vi "插入数据.vi"(8 "error in (no error)":errorcluster, 9 "SQL query":string, 11 "sqlerver in":refnum<class "sqlerver.lvclass">) -> (0 "error out":errorcluster, 3 "sqlerver out":refnum<class "sqlerver.lvclass">)   [LabVIEW 2016, in "sqlerver.lvclass"]
uses:
  sqlerver.lvclass
  sqlerver.lvclass/sqlerver.ctl
  <vilib>/addons/database/Connection.llb/Conn Execute.vi
  <vilib>/addons/database/Recordset.llb/Rec Destroy - Connection.vi
  <vilib>/addons/database/NI_Database_API.lvlib
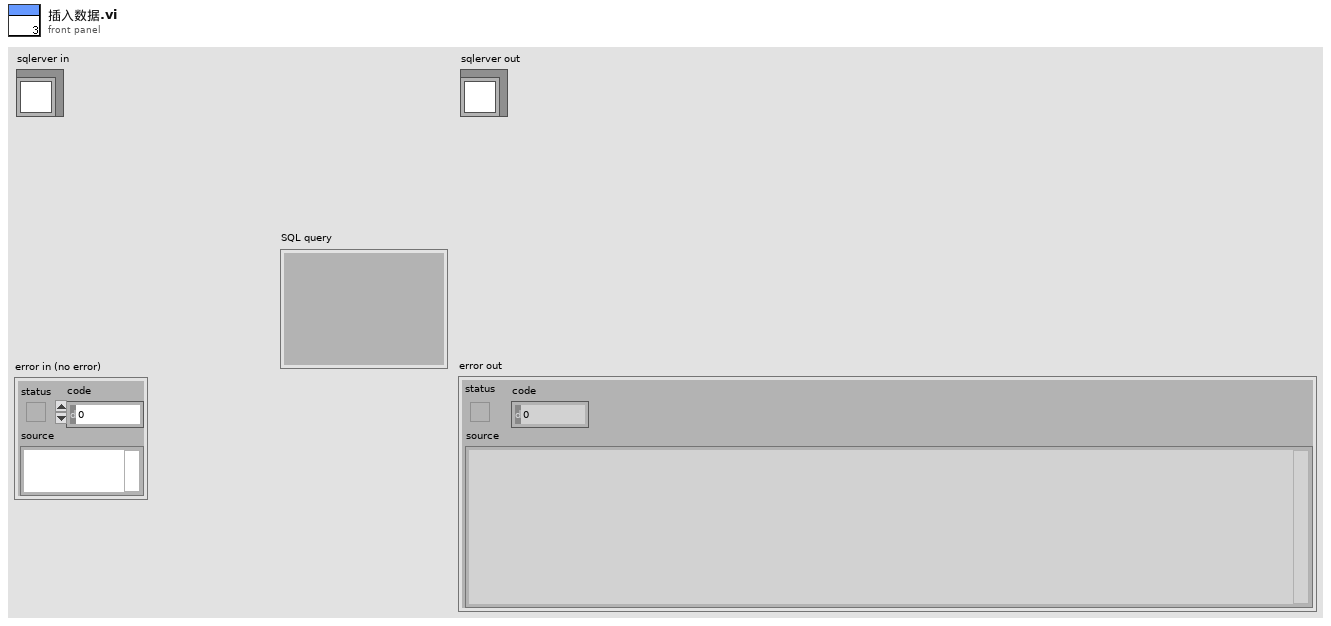
[diagram p1: front panel]
types:
  T1 = typedef "NI_Database_API.lvlib/Conn ObjectReference.ctl" = refnum<k1>
  T2 = typedef "NI_Database_API.lvlib/Rec ObjectReference.ctl" = refnum<k1>
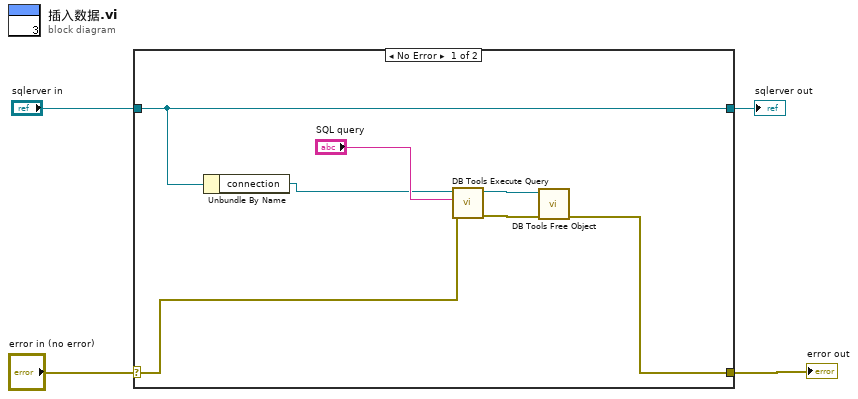
[diagram p0: block diagram]
diagram:
  n1 = case shown="No Error" "error in (no error)" {
    selector: "error in (no error)" -> [w8 w13]
    tunnel: [w7 w13] -> w3
    tunnel: [w6 w12] -> w1
    tunnel: "sqlerver in" -> [w6 w12]
    frame No Error {
      n2 = Unbundle By Name(w6) -> ("connection"=w5:T1)
      n3 = call-poly <vilib>:"DB Tools Execute Query.vi"("error in (no error)"=w8, "SQL query"="SQL query", "connection reference"=w5) -> ("error out"=w10:errorcluster, "recordset reference"=w11:T2)  [unwired: 5 in]
      n4 = call-poly <vilib>:"DB Tools Free Object.vi"("error in (no error)"=w10, "recordset reference"=w11) -> ("error out"=w7:errorcluster)  [unwired: 8 in, 1 out]
    }
    frame Error {
    }
  }
  "error out" <- w3
  "sqlerver out" <- w1
